vi "wsConnectAndAuthenticate.vi"(7 "Access Token":string, 8 "error in (no error)":errorcluster, 10 "Port Name":u16=8123, 11 "Server Address":string="localhost") -> (0 "error out":errorcluster, 1 "Connection Result":string, 2 "Connection Authenticated?":bool, 3 "References":T1)   [LabVIEW 2018, in "HASS-LV-WS_integration.lvlib"]
uses:
  HASS-LV-WS_integration.lvlib
  TypeDef/ReferencesTypeDef.ctl
  TypeDef/QueueTypeDef.ctl
  TypeDef/EventTypeDef.ctl
  TypeDef/registeredEventTypeDef.ctl
  <vilib>/MediaMongrels Ltd/WebSockets/WebSockets/Opcodes.ctl
  <vilib>/MediaMongrels Ltd/WebSockets/WebSockets/WebSockets.lvlib
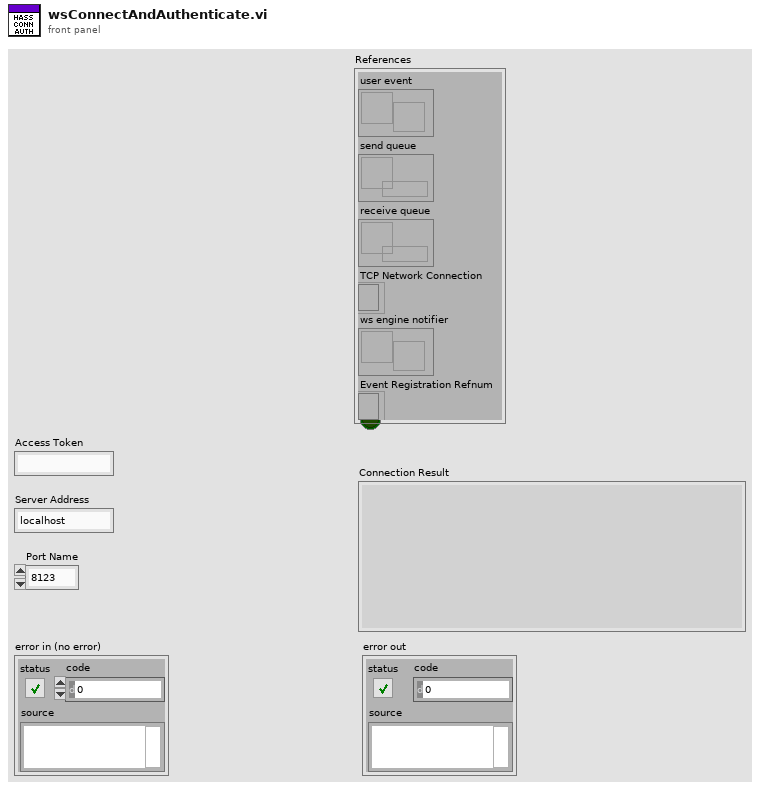
[diagram p1: front panel]
types:
  T1 = typedef "HASS-LV-WS_integration.lvlib/ReferencesTypeDef.ctl" = cluster{"user event":refnum<user-event>, "send queue":refnum<queue>, "receive queue":refnum<queue>, "TCP Network Connection":refnum<k5>, "ws engine notifier ":refnum<notifier>, "Event Registration Refnum":refnum<event-registration>}
  T2 = typedef "HASS-LV-WS_integration.lvlib/registeredEventTypeDef.ctl" = enum16{"Init", "Register", "Unregister", "Get MSG ID", "Get Event Name", "Get All Events"}
  T3 = typedef "HASS-LV-WS_integration.lvlib/EventTypeDef.ctl" = cluster{"Data":variant, "Command":string}
  T4 = typedef "HASS-LV-WS_integration.lvlib/QueueTypeDef.ctl" = cluster{"Data":variant, "Command":string}
  T5 = typedef "WebSockets.lvlib/Opcodes.ctl" = u8
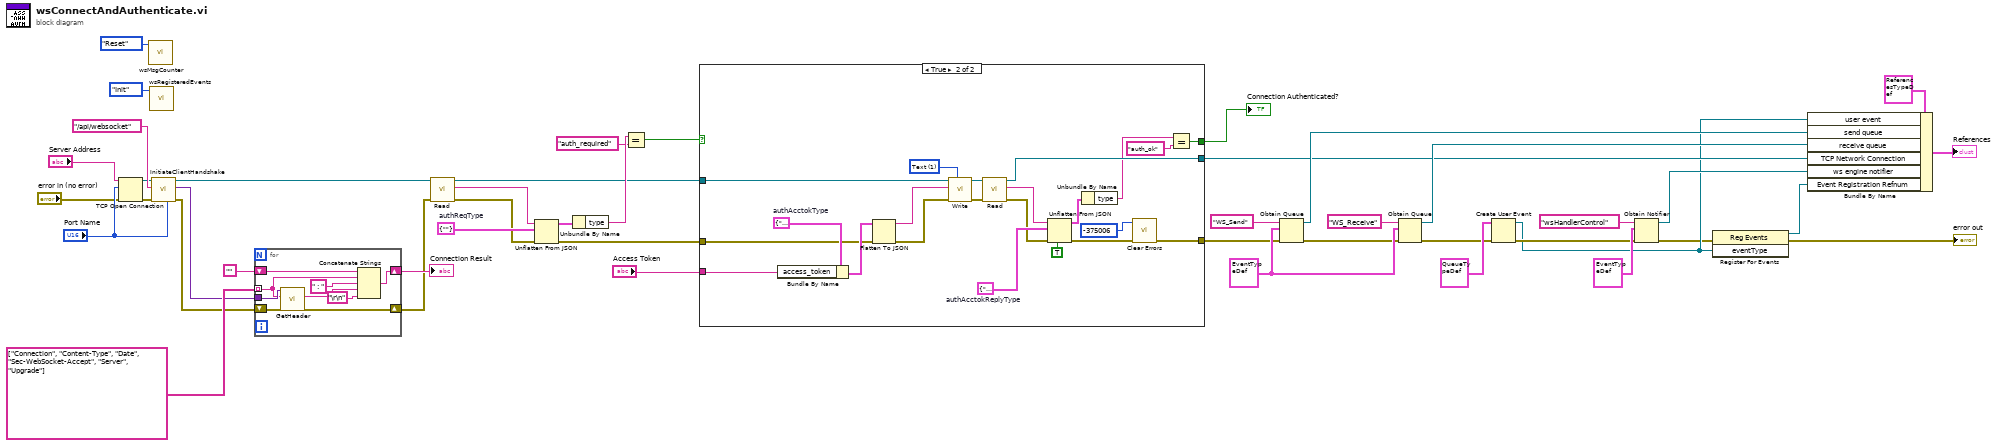
[diagram p0: block diagram]
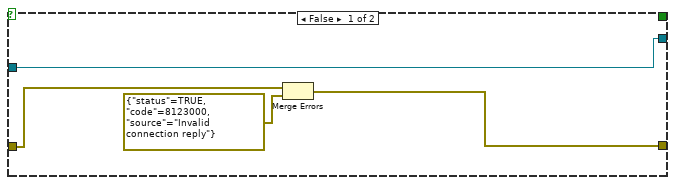
[diagram p2: hidden frame]
diagram:
  w24 = T3 {"Data"=variant, "Command"=""} ("queueType")
  w33 = cluster{"type":string} {"type"=""}  # authReqType
  n1 = TCP Open Connection(address="Server Address", remote port or service name="Port Name", error in (no error)="error in (no error)") -> (connection ID=w35:refnum<k5>, error out=w38:errorcluster)  [unwired: 2 in]
  n2 = call "wsMsgCounter.vi"("Action"=enum16{"Increment", "Reset"}."Reset") -> ()  [unwired: 10 in, 1 out]
  n3 = call "wsRegisteredEvents.vi"("Action"=registeredEventTypeDef."Init") -> ()  [unwired: 7 in, 4 out]
  n4 = call <vilib>:"InitiateClientHandshake.vi"("remote port or service name"="Port Name", "error in (no error)"=w38, "request URI ('/')"="/api/websocket", "WebSocket Connection in"=w35) -> ("error out"=w39:errorcluster, "Return Headers Out"=w37:variant, "WebSocket Connection out"=w43:refnum<k5>)  [unwired: 5 in]
  n5 = for {
    tunnel: w37 -> [w55]
    shift-right: [w53] -> w42
    shift-left: w39 -> [w54]
    tunnel: string[] ["Connection", "Content-Type", "Date", "Sec-WebSocket-Accept", "Server", "Upgrade"] -> [w52] mode=indexing
    shift-right: [w47] -> w45
    shift-left: "" -> [w48]
    n6 = call <vilib>:"GetHeader.vi"("error in (no error)"=w54, "Name"=w52, "Headers In"=w55) -> ("error out"=w53:errorcluster, "Data"=w50:string)  [unwired: 5 in, 2 out]
    n7 = Concatenate Strings(w48, w52, " : " ("string"), w50, "\r\n") -> (w47:string)
  }
  "Connection Result" <- w45
  n8 = call <vilib>:"Read.vi"("error in (no error)"=w42, "WebSocket Connection in"=w43) -> ("error out"=w28:errorcluster, "Data"=w34:string, "WebSocket Connection out"=w27:refnum<k5>)  [unwired: 5 in, 2 out]
  n9 = Unflatten From JSON(JSON string=w34, type and defaults=w33, error in (no error)=w28) -> (value=w32:cluster{"type":string}, error out=w2:errorcluster)  [unwired: 4 in]
  n10 = Unbundle By Name(w32) -> ("type"=w31:string)
  n11 = Equal?(x=w31, y="auth_required") -> (x = y?=w1:bool)
  n12 = case shown="True" w1 {
    tunnel: w2 -> [w59 w77]
    tunnel: [w57 w61] -> w12
    tunnel: "Access Token" -> [_ w79]
    tunnel: w27 -> [w56 w75]
    tunnel: [w56 w71] -> w11
    tunnel: [_ w64] -> w26
    frame False {
      n13 = Merge Errors(w59, errorcluster {"status"=TRUE, "code"=8123000, "source"="Invalid connection reply"} ("error constant")) -> (w57:errorcluster)
    }
    frame True {
      w69 = cluster{"type":string, "message":string} {"type"="", "message"=""}  # authAcctokReplyType
      w78 = T5 1 items=["Cont. Frame"=0, "Text"=1, "Binary"=2, "Close Frame"=8, "Ping"=9, "Pong"=10] ("Opcode (Text)")
      w81 = cluster{"type":string, "access_token":string} {"type"="auth", "access_token"=""}  # authAcctokType
      n14 = Bundle By Name(cluster=w81, "access_token"=w79) -> (w80:cluster{"type":string, "access_token":string})
      n15 = Flatten To JSON(anything=w80, error in (no error)=w77) -> (JSON string=w74:string, 11:w76:errorcluster)  [unwired: 1 in]
      n16 = call <vilib>:"Write.vi"("Opcode (Text)"=w78, "error in (no error)"=w76, "Data"=w74, "WebSocket Connection in"=w75) -> ("error out"=w72:errorcluster, "WebSocket Connection out"=w73:refnum<k5>)  [unwired: 6 in]
      n17 = call <vilib>:"Read.vi"("error in (no error)"=w72, "WebSocket Connection in"=w73) -> ("error out"=w68:errorcluster, "Data"=w70:string, "WebSocket Connection out"=w71:refnum<k5>)  [unwired: 5 in, 2 out]
      n18 = Unflatten From JSON(JSON string=w70, type and defaults=w69, default null elements? (F)=TRUE, error in (no error)=w68) -> (value=w67:cluster{"type":string, "message":string}, error out=w62:errorcluster)  [unwired: 3 in]
      n19 = Unbundle By Name(w67) -> ("type"=w66:string)
      n20 = call <vilib>:"Clear Errors.vi"("error in (no error)"=w62, "specific error code to clear (0: all)"=-375006) -> ("error out"=w61:errorcluster)  [unwired: 4 in, 1 out]
      n21 = Equal?(x=w66, y="auth_ok") -> (x = y?=w64:bool)
    }
  }
  "Connection Authenticated?" <- w26
  n22 = Obtain Queue(name (unnamed)="WS_Send", element data type=w24, error in (no error)=w12) -> (queue out=w18:refnum<queue>, error out=w22:errorcluster)  [unwired: 2 in, 1 out]
  n23 = Obtain Queue(name (unnamed)="WS_Receive", element data type=w24, error in (no error)=w22) -> (queue out=w17:refnum<queue>, error out=w20:errorcluster)  [unwired: 2 in, 1 out]
  n24 = Create User Event(user event datatype=T4 {"Data"=variant, "Command"=""} ("eventType"), error in=w20) -> (user event=w9:refnum<user-event>, error out=w13:errorcluster)
  n25 = Obtain Notifier(name (unnamed)="wsHandlerControl", notification data type=T3 {"Data"=variant, "Command"=""} ("queueType"), error in (no error)=w13) -> (notifier out=w14:refnum<notifier>, error out=w7:errorcluster)  [unwired: 1 in, 1 out]
  n26 = register-events(error in=w7, w9) -> (reference out=w8:refnum<event-registration>, error out=→"error out":errorcluster)  [unwired: 1 in]
  n27 = Bundle By Name(cluster=T1 {"user event"=refnum, "send queue"=refnum, "receive queue"=refnum, "TCP Network Connection"=refnum, "ws engine notifier "=refnum, "Event Registration Refnum"=refnum}, "user event"=w9, "send queue"=w18, "receive queue"=w17, "TCP Network Connection"=w11, "ws engine notifier"=w14, "Event Registration Refnum"=w8) -> (→"References":T1)
